vi "Write refnum.vi"(8 "error in (no error)":errorcluster, 10 "refnum":refnum<file>, 11 "DataWriter in":refnum<class "DataWriter.lvclass">) -> (0 "error out":errorcluster, 3 "DataWriter out":refnum<class "DataWriter.lvclass">)   [LabVIEW 2024, in "Data.lvlib" / "DataWriter.lvclass"]
uses:
  DataWriter.lvclass
  DataWriter.lvclass/DataWriter.ctl
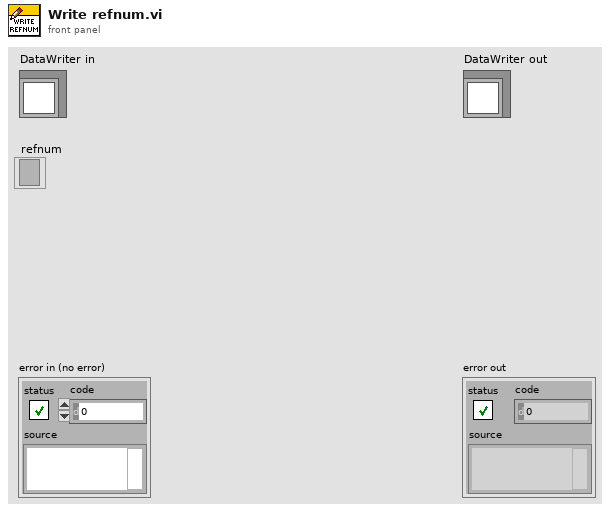
[diagram p1: front panel]
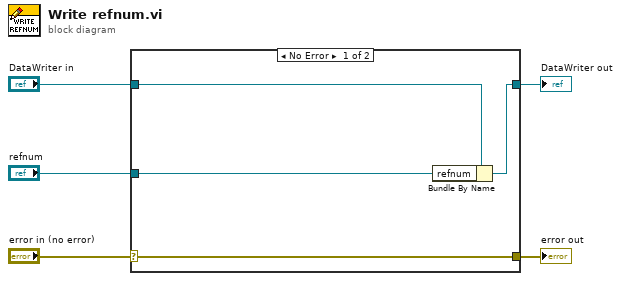
[diagram p0: block diagram]
diagram:
  n1 = case shown="No Error" "error in (no error)" {
    selector: "error in (no error)" -> [w9 w10]
    tunnel: [w9 w10] -> w4
    tunnel: [w7 w11] -> w2
    tunnel: "DataWriter in" -> [w8 w11]
    tunnel: "refnum" -> [w6 _]
    frame No Error {
      n2 = Bundle By Name(cluster=w8, "refnum"=w6) -> (w7:refnum<class "DataWriter.lvclass">)
    }
    frame Error {
    }
  }
  "error out" <- w4
  "DataWriter out" <- w2
